vi "Test App Get Process After Stopping App.vi"(8 "error in (no error)":errorcluster, 11 "Rig Test in":refnum<class "Application Test.lvclass">) -> (0 "error out":errorcluster, 3 "Rig Test out":refnum<class "Application Test.lvclass">)   [LabVIEW 2020, in "Application Test.lvclass"]
uses:
  Application Test.lvclass
  C:/Program Files (x86)/National Instruments/LabVIEW 2020/vi.lib/Asteme/LUnit/Test Case.lvclass
  Framework/Process/Process.lvclass
  Framework/Process/Process.lvclass/Process.ctl
  Framework/Application/Application.lvclass/Application.ctl
  <vilib>/Asteme/LUnit/Test Case.lvclass/Test Case.ctl
  <vilib>/Asteme/LUnit/LUnit Assertion Result.lvclass/LUnit Assertion Result.ctl
  Framework/Application/Private/Add Process to Map.vi
  Framework/Process/Protected/Messaging/Enqueue Message.vi
  Framework/Process/Protected/SubVIs/Set Context.vi
  Framework/Process/Public/Lifecycle/Get Lifecycle State.vi
  Framework/Process/Private/SubVIs/Wait for finish.vi
  Framework/Process/Private/SubVIs/Set Lifecycle State.vi
  Framework/Process/Protected/Messaging/Request Message.vi
  <vilib>/Asteme/LUnit/Palette/Fail.vi
  <vilib>/Asteme/LUnit/Palette/Pass.vi
  <vilib>/Asteme/LUnit/Set Assertion Type.vi
  <vilib>/Utility/error.llb/Clear Errors.vi
  Framework/Process/Community/Leave Process Loop.vi
  Framework/Process/Private/SubVIs/Enqueue Request Message.vi
  <vilib>/Asteme/LUnit/Add test result.vi
  <vilib>/Asteme/LUnit/LUnit Write Passed.vi
  <vilib>/Asteme/LUnit/LUnit Get Test Case.vi
  <vilib>/Asteme/LUnit/Assertion Result/LUnit Get Test Name.vi
  <vilib>/Asteme/LUnit/LUnit Write Message.vi
  <vilib>/Asteme/LUnit/LUnit Write Description.vi
  <vilib>/Asteme/LUnit/LUnit Write Assertion Type.vi
  <vilib>/Asteme/LUnit/Read Test Case Name.vi
  Framework/Application/Application.lvclass
  C:/Users/anton/Documents/GitHub/Triarc-Framework/source/Framework/Process/Process.lvclass
  <vilib>/Utility/error.llb/Error Cluster From Error Code.vi
  Framework/Application/Private/Update Context for Owned Processes.vi
  Framework/Process/Private/SubVIs/Wait for Response Message.vi
  <vilib>/Asteme/LUnit/LUnit Assertion Result.lvclass
  <vilib>/Asteme/LUnit/Test Case.lvclass
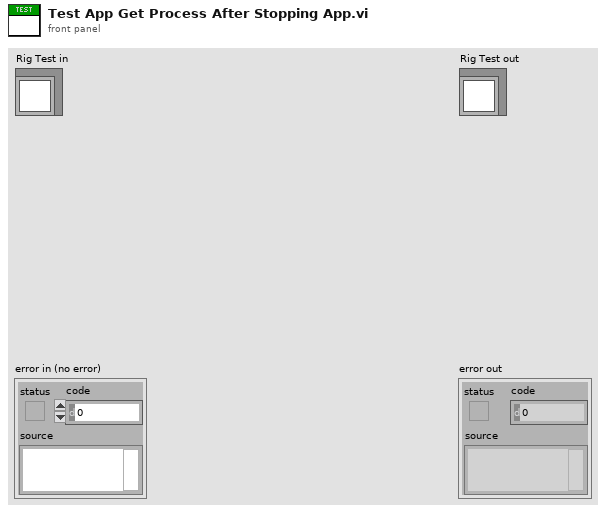
[diagram p1: front panel]
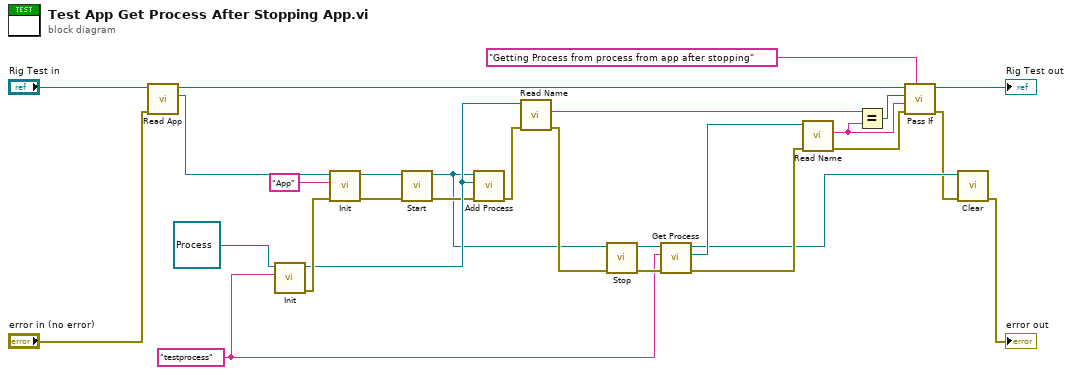
[diagram p0: block diagram]
diagram:
  w2 = "testprocess" ("Name")
  n1 = call "Read App.vi"("error in (no error)"="error in (no error)", "Application Test In"="Rig Test in") -> ("App out"=w27:refnum<class "Application.lvclass">, "Application Test Out"=w19:refnum<class "Application Test.lvclass">)  [unwired: 7 in, 1 out]
  n2 = call-dynamic "Init.vi"("Name"=w2, "Process In"=refnum<class "Process.lvclass"> refnum ("Process.lvclass")) -> ("error out"=w18:errorcluster, "Process Out"=w8:refnum<class "Process.lvclass">)  [unwired: 8 in]
  n3 = call-dynamic "Init.vi"("error in (no error)"=w18, "Name"="App", "Process In"=w27) -> ("error out"=w21:errorcluster, "Process Out"=w5:refnum<class "Application.lvclass">)  [unwired: 7 in]
  n4 = call "Start.vi"("error in (no error)"=w21, "Process In"=w5) -> ("error out"=w6:errorcluster, "Process Out"=w1:refnum<class "Application.lvclass">)  [unwired: 8 in]
  n5 = call "Add Process.vi"("error in (no error)"=w6, "Process"=w8, "Rig In"=w1) -> ("error out"=w4:errorcluster)  [unwired: 7 in, 1 out]
  n6 = call-dynamic "Read Name.vi"("error in (no error)"=w4, "Process In"=w8) -> ("error out"=w3:errorcluster, "Qualified Name"=w7:string)  [unwired: 6 in, 2 out]
  n7 = call "Stop.vi"("error in (no error)"=w3, "Process In"=w1) -> ("error out"=w22:errorcluster, "Process Out"=w23:refnum<class "Application.lvclass">)  [unwired: 7 in, 1 out]
  n8 = call "Get Process.vi"("error in (no error)"=w22, "Process Name"=w2, "Rig In"=w23) -> ("error out"=w13:errorcluster, "App Process"=w16:refnum<class "Process.lvclass">, "Rig Out"=w11:refnum<class "Application.lvclass">)  [unwired: 6 in]
  n9 = call-dynamic "Read Name.vi"("error in (no error)"=w13, "Process In"=w16) -> ("error out"=w12:errorcluster, "Qualified Name"=w14:string)  [unwired: 6 in, 2 out]
  n10 = Equal?(x=w7, y=w14) -> (x = y?=w15:bool)
  n11 = call <vilib>:"Pass If.vi"("Description"="Getting Process from process from app after stopping", "error in (no error)"=w12, "Message"=w14, "Pass?"=w15, "Test Case In"=w19) -> ("error out"=w10:errorcluster, "Test Case Out"=→"Rig Test out":refnum<class "Application Test.lvclass">)  [unwired: 5 in]
  n12 = call-dynamic "Clear.vi"("error in (no error)"=w10, "Application In"=w11) -> ("error out"=→"error out":errorcluster)  [unwired: 8 in, 1 out]
